vi "PXI-4130 Get Channel Indices (RT).vi"(8 "error in (no error)":errorcluster, 11 "Device Item Ref In":T1 format="%.0x") -> (0 "error out":errorcluster, 1 "Read Trigger Index":i32, 2 "Continuous Read? Index":i32, 3 "Device Item Ref Out":T1 format="%.0x")   [LabVIEW 2009, in "PXI-4130 Custom Device.lvlib"]
uses:
  PXI-4130 Custom Device.lvlib
  <vilib>/NI VeriStand/Custom Device API/Custom Device Item Ref.ctl
  PXI-4130 Global Variable.vi
  <vilib>/NI VeriStand/Custom Device API/Custom Device Utility Library.lvlib
  <vilib>/NI VeriStand/Custom Device API/Custom Device API.lvlib
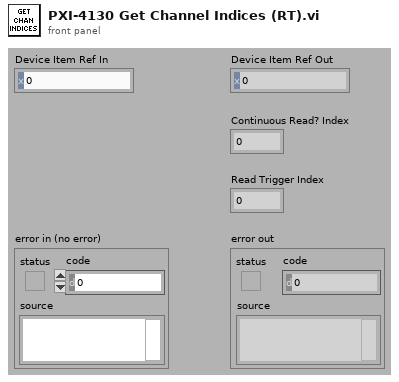
[diagram p1: front panel]
types:
  T1 = typedef "Custom Device API.lvlib/Custom Device Item Ref.ctl" = u64
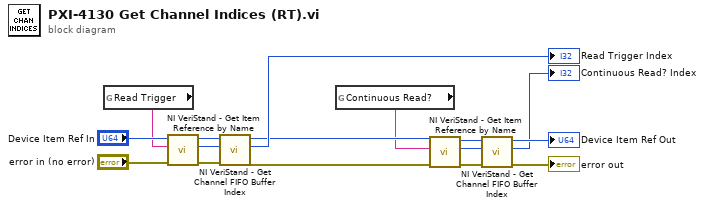
[diagram p0: block diagram]
diagram:
  n1 = global read "PXI-4130 Global Variable.vi" "Read Trigger"() -> (w12:string)
  n2 = call <vilib>:"NI VeriStand - Get Item Reference by Name.vi"("error in (no error)"="error in (no error)", "Item Name"=w12, "Parent Ref in"="Device Item Ref In") -> ("error out"=w10:errorcluster, "Item Ref"=w13:T1, "Parent Ref out"=w14:T1)  [unwired: 5 in, 1 out]
  n3 = call <vilib>:"NI VeriStand - Get Channel FIFO Buffer Index.vi"("error in"=w10, "Channel Ref"=w13, "Device Ref in"=w14) -> ("error out"=w5:errorcluster, "Channel FIFO Buffer Index"=→"Read Trigger Index":i32, "Device Ref out"=w6:T1)  [unwired: 4 in, 2 out]
  n4 = global read "PXI-4130 Global Variable.vi" "Continuous Read?"() -> (w4:string)
  n5 = call <vilib>:"NI VeriStand - Get Item Reference by Name.vi"("error in (no error)"=w5, "Item Name"=w4, "Parent Ref in"=w6) -> ("error out"=w9:errorcluster, "Item Ref"=w8:T1, "Parent Ref out"=w7:T1)  [unwired: 5 in, 1 out]
  n6 = call <vilib>:"NI VeriStand - Get Channel FIFO Buffer Index.vi"("error in"=w9, "Channel Ref"=w8, "Device Ref in"=w7) -> ("error out"=→"error out":errorcluster, "Channel FIFO Buffer Index"=→"Continuous Read? Index":i32, "Device Ref out"=→"Device Item Ref Out":T1)  [unwired: 4 in, 2 out]
